vi "Test JSON to Variant.vi"() -> ()   [LabVIEW 2011]
uses:
  JSON Scalar/JSON Scalar.lvclass
  JSON Value/JSON Value.lvclass
  Variant JSON.lvlib
panel:
  out "String":string
  out "x = y?":bool
  out "data":T1
  in  "Test Cluster":T1={"T2"="test2", "T1"=456.789, "Nest"={"Enum"=enum."AAA", "NestNest"={"A"="Hi", "B"=2.0, "C"=1.0+4.1i}}, "Test Array"=[456.789, 2.0, 3.0], "Boolean"=FALSE, "JSON Scalar.lvclass"=refnum}
  out "JSON String":string
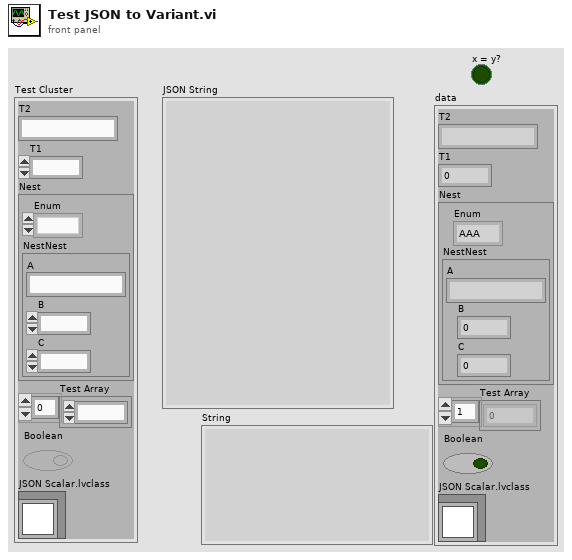
[diagram p1: front panel]
types:
  T1 = cluster{"T2":string, "T1":dbl, "Nest":cluster{"Enum":enum16{"AAA", "BBB", "CCC"}, "NestNest":cluster{"A":string, "B":dbl, "C":cdb}}, "Test Array":dbl[], "Boolean":bool, "JSON Scalar.lvclass":refnum<class "JSON Scalar.lvclass">}
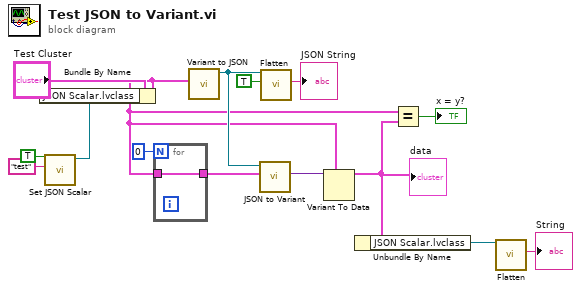
[diagram p0: block diagram]
diagram:
  n1 = call "Set JSON Scalar.vi"("Set as a JSON string (F)"=TRUE, "LabVIEW Text"="test") -> ("JSON Scalar out"=w4:refnum<class "JSON Scalar.lvclass">)  [unwired: 8 in, 1 out]
  n2 = Bundle By Name(cluster="Test Cluster", "JSON Scalar.lvclass"=w4) -> (w5:T1)
  n3 = for {
    N: 0 -> [_]
    tunnel: w5 -> [w16]
    tunnel: [w16] -> w9
  }
  n4 = call "Variant to JSON.vi"("Variant"=w5) -> ("JSON Value out"=w13:refnum<class "JSON Value.lvclass">)  [unwired: 9 in, 1 out]
  n5 = call "JSON to Variant.vi"("Variant (Data Type)"=w9, "JSON Value"=w13) -> ("Variant out"=w12:variant)  [unwired: 8 in, 1 out]
  n6 = call-dynamic "Flatten.vi"("Pretty Print?"=TRUE, "JSON Value in"=w13) -> ("String"=→"JSON String":string)  [unwired: 8 in, 1 out]
  n7 = Variant To Data(type=w5, Variant=w12) -> (data=w3:T1)  [unwired: 1 in, 1 out]
  "data" <- w3
  n8 = Unbundle By Name(w3) -> ("JSON Scalar.lvclass"=w2:refnum<class "JSON Scalar.lvclass">)
  n9 = Equal?(x=w5, y=w3) -> (x = y?=→"x = y?":bool)
  n10 = call-dynamic "Flatten.vi"("JSON Scalar in"=w2) -> ("String"=→"String":string)  [unwired: 9 in, 1 out]
